vi "7.1 Complex Cluster in Array.vi"() -> ()   [LabVIEW 2017]
doc: "### 7.1 Complex Cluster in Array.vi\n\n#### Overview\n\nArray/Cluster nesting is a complex scenario. This example shows API String expression for a complex cluster array. However, this is not a typically recommended usage scenario."
uses:
  8b979ef5-f5f6-4d36-b0d8-cf42d7dfdfe2.vi
  0333efe5-f0fb-4901-b6dd-db031cec30c6.vi
  addons/API-String-Arugments-Support/_Support/Convert API String Arguments to Data(variant).vi
panel:
  out "Retrieve Cluster Array and keep both Type and default value":T1={"String"=["{BoolArray:[0,1,0,1;1,0,1,0;0,1,0,1];Cluster.Boolean:True}", "BoolArray:[TRUE,FALSE,TRUE,FALSE;FALSE,TRUE,FALSE,TRUE;TRUE,FALSE,TRUE,FALSE];Cluster.Boolean:off"], "Reference Cluster Array"=[{"String"="abc", "BoolArray"=[[TRUE, FALSE, TRUE, FALSE], [FALSE, TRUE, FALSE, TRUE], [TRUE, FALSE, TRUE, FALSE]], "Cluster"={"Boolean"=FALSE}}, {"String"="def", "BoolArray"=[[FALSE, TRUE, FALSE, TRUE], [TRUE, FALSE, TRUE, FALSE], [FALSE, TRUE, FALSE, TRUE]], "Cluster"={"Boolean"=TRUE}}], "Retrieved Cluster Array"=[{"String"="abc", "BoolArray"=[[FALSE, TRUE, FALSE, TRUE], [TRUE, FALSE, TRUE, FALSE], [FALSE, TRUE, FALSE, TRUE]], "Cluster"={"Boolean"=TRUE}}, {"String"="def", "BoolArray"=[[TRUE, FALSE, TRUE, FALSE], [FALSE, TRUE, FALSE, TRUE], [TRUE, FALSE, TRUE, FALSE]], "Cluster"={"Boolean"=FALSE}}]}
  out "Retrieve Cluster Array and keep Type Only":T2={"String"="[{BoolArray:[0,1,0,1;1,0,1,0;0,1,0,1];Cluster.Boolean:True},{BoolArray:[TRUE,FALSE,TRUE,FALSE;FALSE,TRUE,FALSE,TRUE;TRUE,FALSE,TRUE,FALSE];Cluster.Boolean:off}]", "Reference Cluster Array"=[{"String"="abc", "BoolArray"=[[TRUE, FALSE, TRUE, FALSE], [FALSE, TRUE, FALSE, TRUE], [TRUE, FALSE, TRUE, FALSE]], "Cluster"={"Boolean"=FALSE}}, {"String"="def", "BoolArray"=[[FALSE, TRUE, FALSE, TRUE], [TRUE, FALSE, TRUE, FALSE], [FALSE, TRUE, FALSE, TRUE]], "Cluster"={"Boolean"=TRUE}}], "Retrieved Cluster Array"=[{"String"="", "BoolArray"=[[FALSE, TRUE, FALSE, TRUE], [TRUE, FALSE, TRUE, FALSE], [FALSE, TRUE, FALSE, TRUE]], "Cluster"={"Boolean"=TRUE}}, {"String"="", "BoolArray"=[[TRUE, FALSE, TRUE, FALSE], [FALSE, TRUE, FALSE, TRUE], [TRUE, FALSE, TRUE, FALSE]], "Cluster"={"Boolean"=FALSE}}]}
  # "#CSM-Example Overview\n\nArray/Cluster nesting is a complex scenario. This example shows API String expression for a complex cluster array. However, this is not a typically recommended usage scenario."
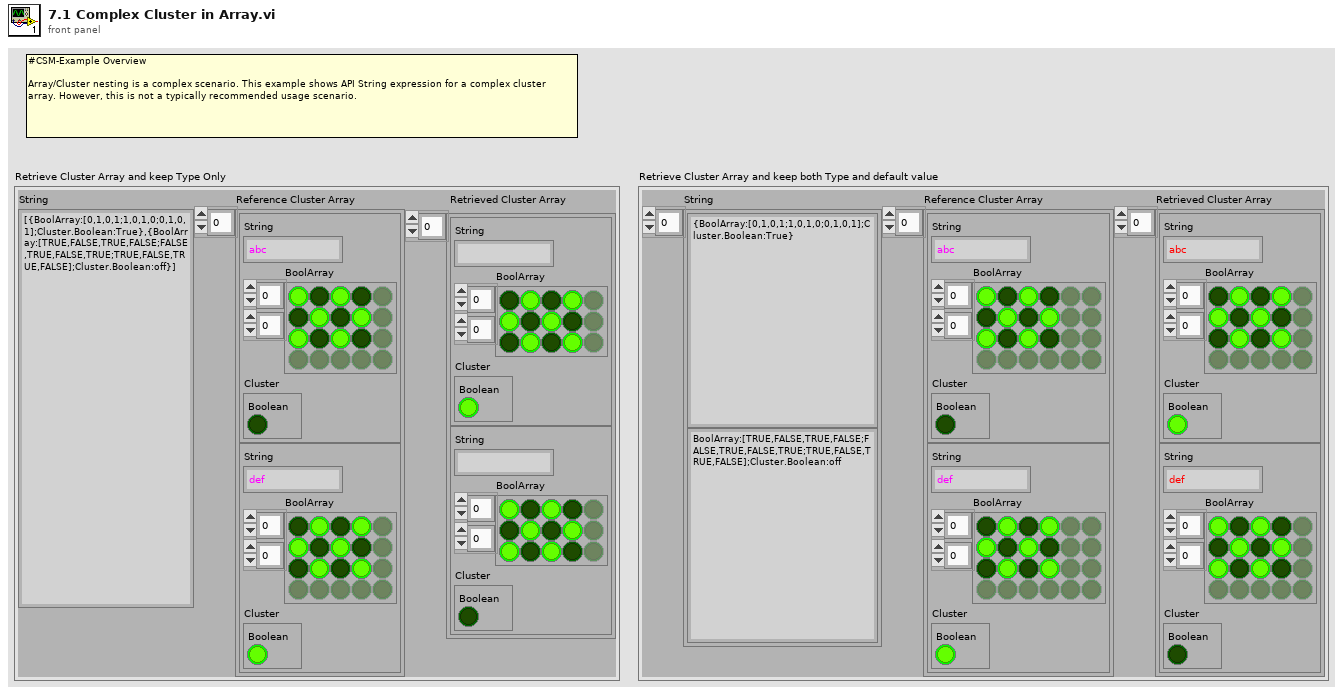
[diagram p1: front panel]
types:
  T1 = cluster{"String":string[], "Reference Cluster Array":cluster{"String":string, "BoolArray":bool[][], "Cluster":cluster{"Boolean":bool}}[], "Retrieved Cluster Array":cluster{"String":string, "BoolArray":bool[][], "Cluster":cluster{"Boolean":bool}}[]}
  T2 = cluster{"String":string, "Reference Cluster Array":cluster{"String":string, "BoolArray":bool[][], "Cluster":cluster{"Boolean":bool}}[], "Retrieved Cluster Array":cluster{"String":string, "BoolArray":bool[][], "Cluster":cluster{"Boolean":bool}}[]}
  T3 = cluster{"String":string, "BoolArray":bool[][], "Cluster":cluster{"Boolean":bool}}[]
  T4 = cluster{"String":string, "Cluster":cluster{"String":string, "BoolArray":bool[][], "Cluster":cluster{"Boolean":bool}}[], "Data":cluster{"String":string, "BoolArray":bool[][], "Cluster":cluster{"Boolean":bool}}[]}
  T5 = cluster{"String":string, "BoolArray":bool[][], "Cluster":cluster{"Boolean":bool}}
  T6 = cluster{"String":string[], "Cluster":cluster{"String":string, "BoolArray":bool[][], "Cluster":cluster{"Boolean":bool}}[], cluster{"String":string, "BoolArray":bool[][], "Cluster":cluster{"Boolean":bool}}[]}
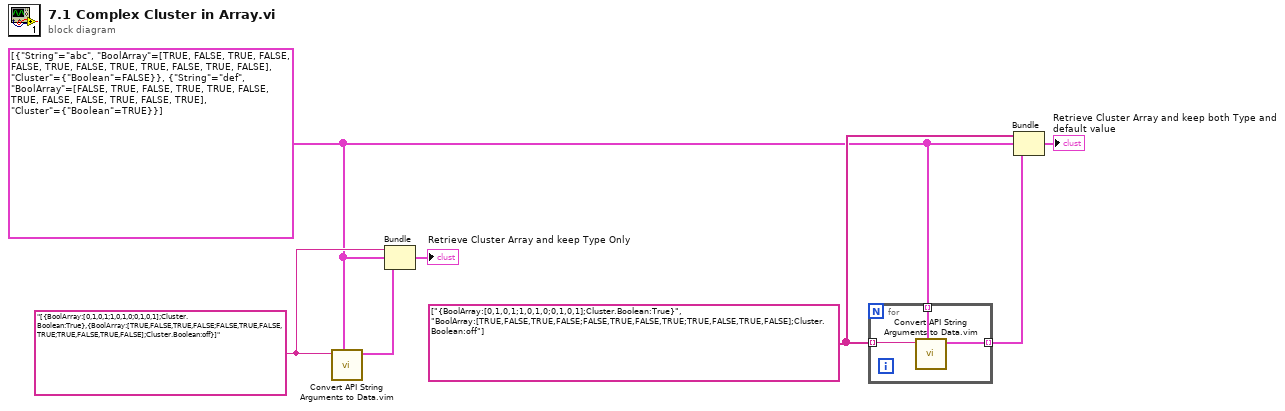
[diagram p0: block diagram]
diagram:
  w4 = string[] ["{BoolArray:[0,1,0,1;1,0,1,0;0,1,0,1];Cluster.Boolean:True}", "BoolArray:[TRUE,FALSE,TRUE,FALSE;FALSE,TRUE,FALSE,TRUE;TRUE,FALSE,TRUE,FALSE];Cluster.Boolean:off"] ("String")
  w5 = "[{BoolArray:[0,1,0,1;1,0,1,0;0,1,0,1];Cluster.Boolean:True},{BoolArray:[TRUE,FALSE,TRUE,FALSE;FALSE,TRUE,FALSE,TRUE;TRUE,FALSE,TRUE,FALSE];Cluster.Boolean:off}]" ("String")
  w3 = T3 [{"String"="abc", "BoolArray"=[[TRUE, FALSE, TRUE, FALSE], [FALSE, TRUE, FALSE, TRUE], [TRUE, FALSE, TRUE, FALSE]], "Cluster"={"Boolean"=FALSE}}, {"String"="def", "BoolArray"=[[FALSE, TRUE, FALSE, TRUE], [TRUE, FALSE, TRUE, FALSE], [FALSE, TRUE, FALSE, TRUE]], "Cluster"={"Boolean"=TRUE}}] ("Cluster")
  n1 = call "Convert API String Arguments to Data.vim"("Reference Type"=w3, "API String"=w5) -> ("Data"=w7:T3)  [unwired: 6 in, 1 out]
  n2 = Bundle("String"=w5, "Cluster"=w3, "Data"=w7) -> (→"Retrieve Cluster Array and keep Type Only":T4)  [unwired: 1 in]
  n3 = for {
    tunnel: w3 -> [w10] mode=indexing
    tunnel: w4 -> [w9] mode=indexing
    tunnel: [w8] -> w2 mode=indexing
    n4 = call "Convert API String Arguments to Data.vim"("Reference Type"=w10, "API String"=w9) -> ("Data"=w8:T5)  [unwired: 6 in, 1 out]
  }
  n5 = Bundle("String"=w4, "Cluster"=w3, w2) -> (→"Retrieve Cluster Array and keep both Type and default value":T6)  [unwired: 1 in]
